vi "BRig_RT_panel_ExpStruct_DAB_v1,10.vi"(7 "input_setValues":bool, 11 "input_dataExp":u16[](array[numeric])) -> (3 "output_dataExp":u16[](array[numeric]))   [LabVIEW 2014]
panel:
  in  "SolenoidProbability_L 2":u16=100 caption="Reward Time [ms]" min=1 max=1000 step=1
  in  "ClosedLoop_LaserHold_l2":bool
  in  "ClosedLoop_LaserHold_l1":bool
  in  "T_CuePenalty":u16=1000 caption="Penalty" min=1 max=10000 step=1
  in  "T_ENLPenalty":u16=100 caption="Penalty" min=10 max=10000 step=10
  in  "LaserSwitch_Probability_L1":u16
  in  "LaserSwitch":u16(slide) max=3 step=1 scale=0.0..3.0
  in  "I_allReward":bool caption="NonSpecific Lick Direction"
  in  "Tcycle_Reward_max_R":u16=1000 caption="Max" min=5 max=5000 step=5
  in  "Tcycle_Reward_min_R":u16=1000 caption="Min" min=5 max=5000 step=5
  in  "Tcycle_Reward_step_R":u16=1000 caption="Penalty" min=1 max=10000 step=1
  in  "Tcycle_Reward_max_L":u16=1000 caption="Max" min=5 max=5000 step=5
  in  "Tcycle_Reward_min_L":u16=1000 caption="Min" min=5 max=5000 step=5
  in  "Tcycle_Reward_step_L":u16=1000 caption="Penalty" min=1 max=10000 step=1
  in  "T_Cue_LED_max":u16=1000 caption="Max" min=5 max=5000 step=5
  in  "T_Cue_LED_min":u16=1000 caption="Min" min=5 max=5000 step=5
  in  "T_Cue_LED_step":u16=1000 caption="Penalty" min=1 max=10000 step=1
  in  "SolenoidProbability_L":u16=100 caption="Reward Time [ms]" min=1 max=1000 step=1
  in  "SolenoidProbability_R":u16=100 caption="Reward Time [ms]" min=1 max=1000 step=1
  in  "T_Cue_Audio_max":u16=1000 caption="Max" min=5 max=5000 step=5
  in  "T_Cue_Audio_min":u16=1000 caption="Min" min=5 max=5000 step=5
  in  "Tcycle_Timeout":u16=1000 caption="Timeout Time [ms]" min=10 max=10000 step=1
  in  "Tcycle_Selection":u16=1000 caption="Answer Time [ms]" min=1 max=10000 step=1
  in  "Tcycle_RewardPost":u16=1000 caption="Consumption Time [ms]" min=250 max=10000 step=250
  in  "T_Cue_Audio_step":u16=1000 caption="Penalty" min=1 max=10000 step=1
  in  "T_ENL_step":u16=100 caption="Penalty" min=10 max=10000 step=10
  in  "T_ENL_max":u16=1000 caption="Max" min=250 max=10000 step=250
  in  "T_ENL_min":u16=1000 caption="Min" min=250 max=10000 step=250
  # "Experiment Task Structure"
  # "(Laser1 or Laser2)\nLaser1 probability"
  # "Min            Max               Step        Penalty"
  # "Enforced\nNonLick"
  # "(ClosedLoop Structure)"
  # "Hold Laser1"
  # "Hold Laser2"
  # "Cue Audio"
  # "Cue LED"
  # "Selection"
  # "Reward - Dispense Water"
  # "Min            Max            StepSize"
  # "Flip Directionality\nAfter X trials\n(Flip Reward Amount and Prob)"
  # "Left"
  # "Right"
  # "Dispense Water Probability"
  # "%"
  # "Left"
  # "Right"
  # "%"
  # "Reward - Consumption"
  # "Penalty - Choice Timeout"
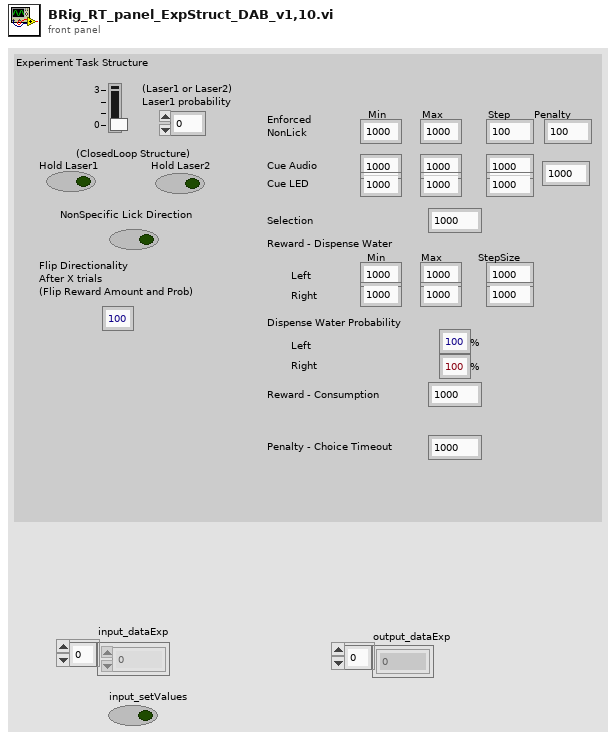
[diagram p1: front panel]
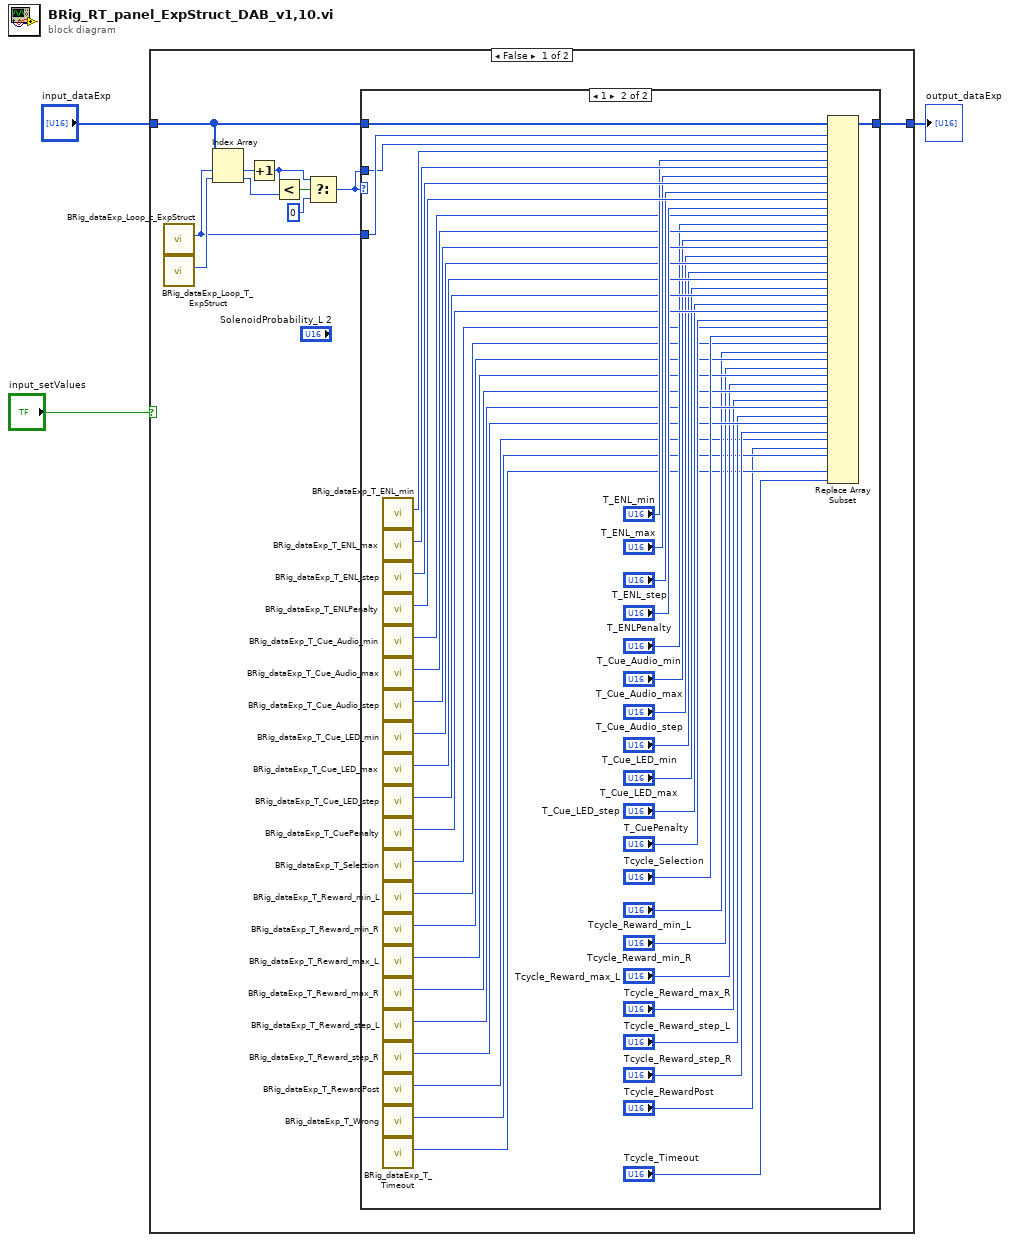
[diagram p0: block diagram]
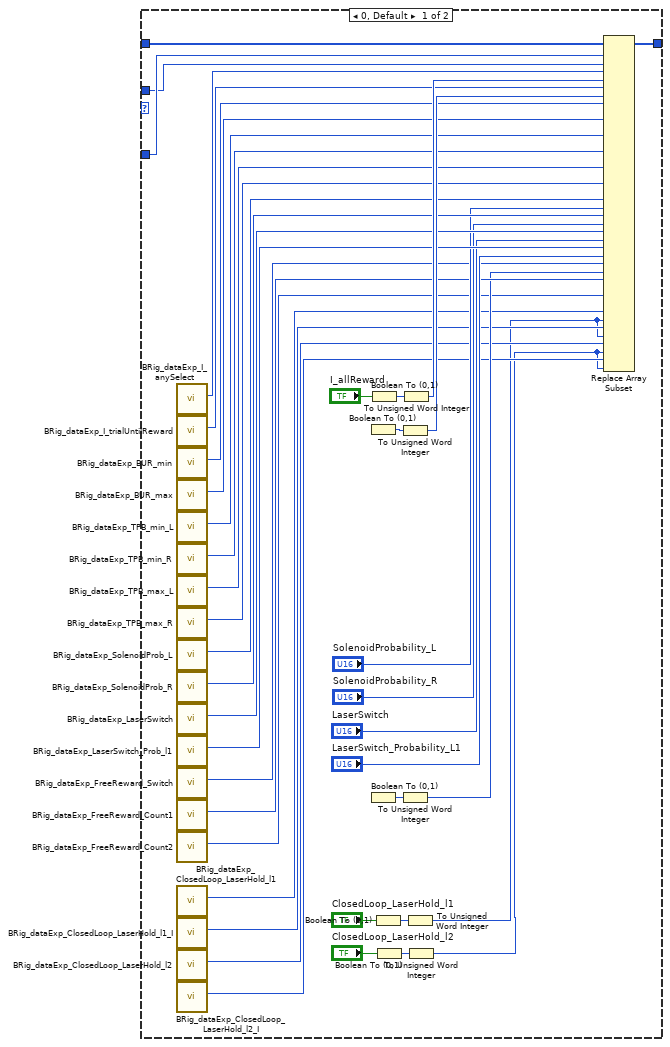
[diagram p2: hidden frame]
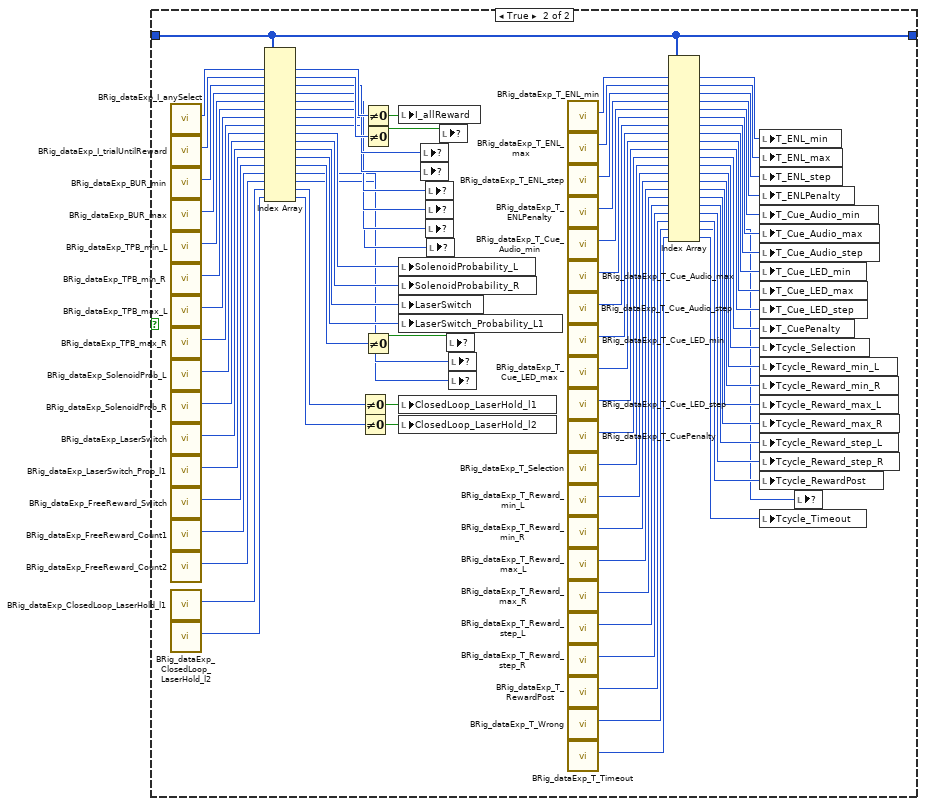
[diagram p3: hidden frame]
diagram:
  n1 = case shown="False" "input_setValues" {
    tunnel: [w13 w158] -> w3
    tunnel: "input_dataExp" -> [w12 w158]
    frame False {
      n2 = call "BRig_dataExp_Loop_c_ExpStruct.vi"() -> ("output_Loop_c_ExpStruct"=w6:i32)  [unwired: 11 in]
      n3 = call "BRig_dataExp_Loop_T_ExpStruct.vi"() -> ("output_Loop_T_ExpStruct"=w11:i32)  [unwired: 11 in]
      n4 = Index Array(array=w12, index #1=w6, index #2=w11) -> (element #1=w10:u16, element #2=w9:u16)
      n5 = Increment(x=w10) -> (x+1=w5:u16)
      n6 = Less?(x=w5, y=w9) -> (x < y?=w8:bool)
      n7 = Select(t=w5, s=w8, f=u16 0) -> (s? t:f=w4:u16)
      n8 = case shown="1" w4 {
        tunnel: w12 -> [w61 w107]
        tunnel: [w60 w106] -> w13
        tunnel: w6 -> [w32 w105]
        tunnel: w4 -> [w31 w104]
        frame 0, Default {
          n9 = call "BRig_dataExp_I_anySelect.vi"() -> ("output_I_anySelect"=w59:i32)  [unwired: 11 in]
          n10 = call "BRig_dataExp_I_trialUntilReward.vi"() -> ("output_I_trialUntilReward"=w55:i32)  [unwired: 11 in]
          n11 = call "BRig_dataExp_BUR_min.vi"() -> ("output_BUR_min"=w52:i32)  [unwired: 11 in]
          n12 = call "BRig_dataExp_BUR_max.vi"() -> ("output_BUR_max"=w51:i32)  [unwired: 11 in]
          n13 = call "BRig_dataExp_TPB_min_L.vi"() -> ("output_TPB_min_L"=w48:i32)  [unwired: 11 in]
          n14 = call "BRig_dataExp_TPB_min_R.vi"() -> ("output_TPB_min_R"=w47:i32)  [unwired: 11 in]
          n15 = call "BRig_dataExp_TPB_max_L.vi"() -> ("output_TPB_max_L"=w46:i32)  [unwired: 11 in]
          n16 = call "BRig_dataExp_TPB_max_R.vi"() -> ("output_TPB_max_R"=w45:i32)  [unwired: 11 in]
          n17 = call "BRig_dataExp_SolenoidProb_L.vi"() -> ("output_SolenoidProbability_L"=w40:i32)  [unwired: 11 in]
          n18 = call "BRig_dataExp_SolenoidProb_R.vi"() -> ("output_SolenoidProbability_R"=w39:i32)  [unwired: 11 in]
          n19 = call "BRig_dataExp_LaserSwitch.vi"() -> ("output_LaserSwitch"=w38:i32)  [unwired: 11 in]
          n20 = call "BRig_dataExp_LaserSwitch_Prob_l1.vi"() -> ("output_LaserSwitch_Probability_L1"=w37:i32)  [unwired: 11 in]
          n21 = call "BRig_dataExp_FreeReward_Switch.vi"() -> ("output_FreeReward_Switch"=w29:i32)  [unwired: 11 in]
          n22 = call "BRig_dataExp_FreeReward_Count1.vi"() -> ("output_FreeReward_Count"=w28:i32)  [unwired: 11 in]
          n23 = call "BRig_dataExp_FreeReward_Count2.vi"() -> ("output_FreeReward_Count"=w25:i32)  [unwired: 11 in]
          n24 = call "BRig_dataExp_ClosedLoop_LaserHold_l1.vi"() -> ("output_CloseLoop_LaserHold_l1"=w23:i32)  [unwired: 11 in]
          n25 = call "BRig_dataExp_ClosedLoop_LaserHold_l1_I.vi"() -> ("output_CloseLoop_LaserHold_l1_I"=w22:i32)  [unwired: 11 in]
          n26 = call "BRig_dataExp_ClosedLoop_LaserHold_l2.vi"() -> ("output_CloseLoop_LaserHold_l2"=w21:i32)  [unwired: 11 in]
          n27 = call "BRig_dataExp_ClosedLoop_LaserHold_l2_I.vi"() -> ("output_CloseLoop_LaserHold_l2_I"=w20:i32)  [unwired: 11 in]
          n28 = Boolean To (0,1)() -> (0, 1=w54:i16)  [unwired: 1 in]
          n29 = Boolean To (0,1)() -> (0, 1=w30:i16)  [unwired: 1 in]
          n30 = Boolean To (0,1)(Boolean="I_allReward") -> (0, 1=w57:i16)
          n31 = Boolean To (0,1)(Boolean="ClosedLoop_LaserHold_l1") -> (0, 1=w19:i16)
          n32 = Boolean To (0,1)(Boolean="ClosedLoop_LaserHold_l2") -> (0, 1=w17:i16)
          n33 = To Unsigned Word Integer(number=w54) -> (unsigned 16bit integer=w53:u16)
          n34 = To Unsigned Word Integer(number=w30) -> (unsigned 16bit integer=w27:u16)
          n35 = To Unsigned Word Integer(number=w57) -> (unsigned 16bit integer=w56:u16)
          n36 = To Unsigned Word Integer(number=w19) -> (unsigned 16bit integer=w15:u16)
          n37 = To Unsigned Word Integer(number=w17) -> (unsigned 16bit integer=w14:u16)
          n38 = Replace Array Subset(array=w61, new element #1=w31, index #1=w32, new element #2=w56, index #2=w59, new element #3=w53, index #3=w55, index #4=w52, index #5=w51, index #6=w48, index #7=w47, index #8=w46, index #9=w45, new element #10="SolenoidProbability_L", index #10=w40, new element #11="SolenoidProbability_R", index #11=w39, new element #12="LaserSwitch", index #12=w38, new element #13="LaserSwitch_Probability_L1", index #13=w37, new element #14=w27, index #14=w29, index #15=w28, index #16=w25, new element #17=w15, index #17=w23, new element #18=w15, index #18=w22, new element #19=w14, index #19=w21, new element #20=w14, index #20=w20) -> (w60:u16[], new element #4=w50:u16, new element #5=w49:u16, new element #6=w44:u16, new element #7=w43:u16, new element #8=w42:u16, new element #9=w41:u16, new element #15=w26:u16, new element #16=w24:u16)
        }
        frame 1 {
          n39 = call "BRig_dataExp_T_ENL_min.vi"() -> ("output_T_ENL_min"=w103:i32)  [unwired: 11 in]
          n40 = call "BRig_dataExp_T_ENL_max.vi"() -> ("output_T_ENL_max"=w102:i32)  [unwired: 11 in]
          n41 = call "BRig_dataExp_T_ENL_step.vi"() -> ("output_T_ENL_step"=w101:i32)  [unwired: 11 in]
          n42 = call "BRig_dataExp_T_ENLPenalty.vi"() -> ("output_ENL_penalty"=w100:i32)  [unwired: 11 in]
          n43 = call "BRig_dataExp_T_Cue_Audio_min.vi"() -> ("output_T_Cue_Audio_min"=w95:i32)  [unwired: 11 in]
          n44 = call "BRig_dataExp_T_Cue_Audio_max.vi"() -> ("output_T_Cue_Audio_max"=w94:i32)  [unwired: 11 in]
          n45 = call "BRig_dataExp_T_Cue_Audio_step.vi"() -> ("output_T_Cue_Audio_step"=w93:i32)  [unwired: 11 in]
          n46 = call "BRig_dataExp_T_Cue_LED_min.vi"() -> ("output_T_Cue_LED_min"=w92:i32)  [unwired: 11 in]
          n47 = call "BRig_dataExp_T_Cue_LED_max.vi"() -> ("output_T_Cue_LED_max"=w91:i32)  [unwired: 11 in]
          n48 = call "BRig_dataExp_T_Cue_LED_step.vi"() -> ("output_T_Cue_LED_step"=w90:i32)  [unwired: 11 in]
          n49 = call "BRig_dataExp_T_CuePenalty.vi"() -> ("output_T_CuePenalty"=w89:i32)  [unwired: 11 in]
          n50 = call "BRig_dataExp_T_Selection.vi"() -> ("output_T_Selection"=w81:i32)  [unwired: 11 in]
          n51 = call "BRig_dataExp_T_Reward_min_L.vi"() -> ("output_Tcycle_Reward_min_L"=w79:i32)  [unwired: 11 in]
          n52 = call "BRig_dataExp_T_Reward_min_R.vi"() -> ("output_T_Reward_min_R"=w78:i32)  [unwired: 11 in]
          n53 = call "BRig_dataExp_T_Reward_max_L.vi"() -> ("output_T_Reward_max_L"=w77:i32)  [unwired: 11 in]
          n54 = call "BRig_dataExp_T_Reward_max_R.vi"() -> ("output_T_Reward_max_R"=w76:i32)  [unwired: 11 in]
          n55 = call "BRig_dataExp_T_Reward_step_L.vi"() -> ("output_T_Reward_step_L"=w75:i32)  [unwired: 11 in]
          n56 = call "BRig_dataExp_T_Reward_step_R.vi"() -> ("output_T_Reward_step_R"=w74:i32)  [unwired: 11 in]
          n57 = call "BRig_dataExp_T_RewardPost.vi"() -> ("output_T_RewardPost"=w67:i32)  [unwired: 11 in]
          n58 = call "BRig_dataExp_T_Wrong.vi"() -> ("output_T_Wrong"=w66:i32)  [unwired: 11 in]
          n59 = call "BRig_dataExp_T_Timeout.vi"() -> ("output_T_Timeout"=w65:i32)  [unwired: 11 in]
          n60 = Replace Array Subset(array=w107, new element #1=w104, index #1=w105, new element #2="T_ENL_min", index #2=w103, new element #3="T_ENL_max", index #3=w102, new element #4="T_ENL_step", index #4=w101, new element #5="T_ENLPenalty", index #5=w100, new element #6="T_Cue_Audio_min", index #6=w95, new element #7="T_Cue_Audio_max", index #7=w94, new element #8="T_Cue_Audio_step", index #8=w93, new element #9="T_Cue_LED_min", index #9=w92, new element #10="T_Cue_LED_max", index #10=w91, new element #11="T_Cue_LED_step", index #11=w90, new element #12="T_CuePenalty", index #12=w89, new element #13="Tcycle_Selection", index #13=w81, new element #14="Tcycle_Reward_min_L", index #14=w79, new element #15="Tcycle_Reward_min_R", index #15=w78, new element #16="Tcycle_Reward_max_L", index #16=w77, new element #17="Tcycle_Reward_max_R", index #17=w76, new element #18="Tcycle_Reward_step_L", index #18=w75, new element #19="Tcycle_Reward_step_R", index #19=w74, new element #20="Tcycle_RewardPost", index #20=w67, index #21=w66, new element #22="Tcycle_Timeout", index #22=w65) -> (w106:u16[], new element #21=w63:u16)
        }
      }
    }
    frame True {
      n61 = call "BRig_dataExp_I_anySelect.vi"() -> ("output_I_anySelect"=w189:i32)  [unwired: 11 in]
      n62 = call "BRig_dataExp_I_trialUntilReward.vi"() -> ("output_I_trialUntilReward"=w188:i32)  [unwired: 11 in]
      n63 = call "BRig_dataExp_BUR_min.vi"() -> ("output_BUR_min"=w187:i32)  [unwired: 11 in]
      n64 = call "BRig_dataExp_BUR_max.vi"() -> ("output_BUR_max"=w186:i32)  [unwired: 11 in]
      n65 = call "BRig_dataExp_TPB_min_L.vi"() -> ("output_TPB_min_L"=w185:i32)  [unwired: 11 in]
      n66 = call "BRig_dataExp_TPB_min_R.vi"() -> ("output_TPB_min_R"=w184:i32)  [unwired: 11 in]
      n67 = call "BRig_dataExp_TPB_max_L.vi"() -> ("output_TPB_max_L"=w183:i32)  [unwired: 11 in]
      n68 = call "BRig_dataExp_TPB_max_R.vi"() -> ("output_TPB_max_R"=w182:i32)  [unwired: 11 in]
      n69 = call "BRig_dataExp_SolenoidProb_L.vi"() -> ("output_SolenoidProbability_L"=w181:i32)  [unwired: 11 in]
      n70 = call "BRig_dataExp_SolenoidProb_R.vi"() -> ("output_SolenoidProbability_R"=w180:i32)  [unwired: 11 in]
      n71 = call "BRig_dataExp_LaserSwitch.vi"() -> ("output_LaserSwitch"=w179:i32)  [unwired: 11 in]
      n72 = call "BRig_dataExp_LaserSwitch_Prob_l1.vi"() -> ("output_LaserSwitch_Probability_L1"=w178:i32)  [unwired: 11 in]
      n73 = call "BRig_dataExp_FreeReward_Switch.vi"() -> ("output_FreeReward_Switch"=w177:i32)  [unwired: 11 in]
      n74 = call "BRig_dataExp_FreeReward_Count1.vi"() -> ("output_FreeReward_Count"=w176:i32)  [unwired: 11 in]
      n75 = call "BRig_dataExp_FreeReward_Count2.vi"() -> ("output_FreeReward_Count"=w115:i32)  [unwired: 11 in]
      n76 = call "BRig_dataExp_ClosedLoop_LaserHold_l1.vi"() -> ("output_CloseLoop_LaserHold_l1"=w113:i32)  [unwired: 11 in]
      n77 = call "BRig_dataExp_ClosedLoop_LaserHold_l2.vi"() -> ("output_CloseLoop_LaserHold_l2"=w112:i32)  [unwired: 11 in]
      n78 = Index Array(array=w158, index #1=w189, index #2=w188, index #3=w187, index #4=w186, index #5=w185, index #6=w184, index #7=w183, index #8=w182, index #9=w181, index #10=w180, index #11=w179, index #12=w178, index #13=w177, index #14=w176, index #15=w115, index #16=w113, index #17=w112) -> (element #1=w172:u16, element #2=w171:u16, element #3=w170:u16, element #4=w169:u16, element #5=w168:u16, element #6=w167:u16, element #7=w166:u16, element #8=w165:u16, element #9=w164:u16, element #10=w163:u16, element #11=w162:u16, element #12=w161:u16, element #13=w160:u16, element #14=w159:u16, element #15=w114:u16, element #16=w109:u16, element #17=w108:u16)
      n79 = Not Equal To 0?(x=w109) -> (x != 0?=w111:bool)
      n80 = Not Equal To 0?(x=w108) -> (x != 0?=w110:bool)
      n81 = Not Equal To 0?(x=w172) -> (x != 0?=w175:bool)
      n82 = Not Equal To 0?(x=w171) -> (x != 0?=w174:bool)
      n83 = Not Equal To 0?(x=w160) -> (x != 0?=w173:bool)
      n84 = local write "I_allReward"(w175) -> ()
      n85 = local write "SolenoidProbability_L"(w164) -> ()
      n86 = local write "SolenoidProbability_R"(w163) -> ()
      n87 = local write "LaserSwitch"(w162) -> ()
      n88 = local write "LaserSwitch_Probability_L1"(w161) -> ()
      n89 = local write "ClosedLoop_LaserHold_l1"(w111) -> ()
      n90 = local write "ClosedLoop_LaserHold_l2"(w110) -> ()
      n91 = local write item#-1(w170) -> ()
      n92 = local write item#-1(w169) -> ()
      n93 = local write item#-1(w168) -> ()
      n94 = local write item#-1(w167) -> ()
      n95 = local write item#-1(w166) -> ()
      n96 = local write item#-1(w165) -> ()
      n97 = local write item#-1(w174) -> ()
      n98 = local write item#-1(w173) -> ()
      n99 = local write item#-1(w159) -> ()
      n100 = local write item#-1(w114) -> ()
      n101 = call "BRig_dataExp_T_ENL_min.vi"() -> ("output_T_ENL_min"=w157:i32)  [unwired: 11 in]
      n102 = call "BRig_dataExp_T_ENL_max.vi"() -> ("output_T_ENL_max"=w156:i32)  [unwired: 11 in]
      n103 = call "BRig_dataExp_T_ENL_step.vi"() -> ("output_T_ENL_step"=w155:i32)  [unwired: 11 in]
      n104 = call "BRig_dataExp_T_ENLPenalty.vi"() -> ("output_ENL_penalty"=w154:i32)  [unwired: 11 in]
      n105 = call "BRig_dataExp_T_Cue_Audio_min.vi"() -> ("output_T_Cue_Audio_min"=w153:i32)  [unwired: 11 in]
      n106 = call "BRig_dataExp_T_Cue_Audio_max.vi"() -> ("output_T_Cue_Audio_max"=w152:i32)  [unwired: 11 in]
      n107 = call "BRig_dataExp_T_Cue_Audio_step.vi"() -> ("output_T_Cue_Audio_step"=w151:i32)  [unwired: 11 in]
      n108 = call "BRig_dataExp_T_Cue_LED_min.vi"() -> ("output_T_Cue_LED_min"=w150:i32)  [unwired: 11 in]
      n109 = call "BRig_dataExp_T_Cue_LED_max.vi"() -> ("output_T_Cue_LED_max"=w149:i32)  [unwired: 11 in]
      n110 = call "BRig_dataExp_T_Cue_LED_step.vi"() -> ("output_T_Cue_LED_step"=w148:i32)  [unwired: 11 in]
      n111 = call "BRig_dataExp_T_CuePenalty.vi"() -> ("output_T_CuePenalty"=w147:i32)  [unwired: 11 in]
      n112 = call "BRig_dataExp_T_Selection.vi"() -> ("output_T_Selection"=w146:i32)  [unwired: 11 in]
      n113 = call "BRig_dataExp_T_Reward_min_L.vi"() -> ("output_Tcycle_Reward_min_L"=w145:i32)  [unwired: 11 in]
      n114 = call "BRig_dataExp_T_Reward_min_R.vi"() -> ("output_T_Reward_min_R"=w144:i32)  [unwired: 11 in]
      n115 = call "BRig_dataExp_T_Reward_max_L.vi"() -> ("output_T_Reward_max_L"=w143:i32)  [unwired: 11 in]
      n116 = call "BRig_dataExp_T_Reward_max_R.vi"() -> ("output_T_Reward_max_R"=w142:i32)  [unwired: 11 in]
      n117 = call "BRig_dataExp_T_Reward_step_L.vi"() -> ("output_T_Reward_step_L"=w141:i32)  [unwired: 11 in]
      n118 = call "BRig_dataExp_T_Reward_step_R.vi"() -> ("output_T_Reward_step_R"=w140:i32)  [unwired: 11 in]
      n119 = call "BRig_dataExp_T_RewardPost.vi"() -> ("output_T_RewardPost"=w139:i32)  [unwired: 11 in]
      n120 = call "BRig_dataExp_T_Wrong.vi"() -> ("output_T_Wrong"=w138:i32)  [unwired: 11 in]
      n121 = call "BRig_dataExp_T_Timeout.vi"() -> ("output_T_Timeout"=w137:i32)  [unwired: 11 in]
      n122 = Index Array(array=w158, index #1=w157, index #2=w156, index #3=w155, index #4=w154, index #5=w153, index #6=w152, index #7=w151, index #8=w150, index #9=w149, index #10=w148, index #11=w147, index #12=w146, index #13=w145, index #14=w144, index #15=w143, index #16=w142, index #17=w141, index #18=w140, index #19=w139, index #20=w138, index #21=w137) -> (element #1=w136:u16, element #2=w135:u16, element #3=w134:u16, element #4=w133:u16, element #5=w132:u16, element #6=w131:u16, element #7=w130:u16, element #8=w129:u16, element #9=w128:u16, element #10=w127:u16, element #11=w126:u16, element #12=w125:u16, element #13=w124:u16, element #14=w123:u16, element #15=w122:u16, element #16=w121:u16, element #17=w120:u16, element #18=w119:u16, element #19=w118:u16, element #20=w117:u16, element #21=w116:u16)
      n123 = local write "T_ENL_min"(w136) -> ()
      n124 = local write "T_ENL_max"(w135) -> ()
      n125 = local write "T_ENL_step"(w134) -> ()
      n126 = local write "T_ENLPenalty"(w133) -> ()
      n127 = local write "T_Cue_Audio_min"(w132) -> ()
      n128 = local write "T_Cue_Audio_max"(w131) -> ()
      n129 = local write "T_Cue_Audio_step"(w130) -> ()
      n130 = local write "T_Cue_LED_min"(w129) -> ()
      n131 = local write "T_Cue_LED_max"(w128) -> ()
      n132 = local write "T_Cue_LED_step"(w127) -> ()
      n133 = local write "T_CuePenalty"(w126) -> ()
      n134 = local write "Tcycle_Selection"(w125) -> ()
      n135 = local write "Tcycle_Reward_min_L"(w124) -> ()
      n136 = local write "Tcycle_Reward_min_R"(w123) -> ()
      n137 = local write "Tcycle_Reward_max_L"(w122) -> ()
      n138 = local write "Tcycle_Reward_max_R"(w121) -> ()
      n139 = local write "Tcycle_Reward_step_L"(w120) -> ()
      n140 = local write "Tcycle_Reward_step_R"(w119) -> ()
      n141 = local write "Tcycle_RewardPost"(w118) -> ()
      n142 = local write "Tcycle_Timeout"(w116) -> ()
      n143 = local write item#-1(w117) -> ()
    }
  }
  "output_dataExp" <- w3
